vi "Source Voltage PPMU.vi"(8 "error in (no error)":errorcluster, 9 "voltage level":dbl, 10 "All Pins":string[](array[string]), 11 "Semiconductor Module Context":T1) -> (0 "error out":errorcluster, 3 "voltage measurements":dbl[][](array[numeric]))   [LabVIEW 2013]
uses:
  <vilib>/NI_TestStand_SemiconductorModule/NI_TestStand_Semiconductor_Module.lvlibp/PinMap/General/SemiconductorModuleContext.ctl
  <vilib>/NI_TestStand_SemiconductorModule/NI_TestStand_Semiconductor_Module.lvlibp/PinMap/General/NIInstrumentTypeIDs.ctl
  <vilib>/NI_TestStand_SemiconductorModule/NI_TestStand_Semiconductor_Module.lvlibp/PinMap/HSDIO/PinsToNIHSDIOSessions.vi
  <vilib>/NI_TestStand_SemiconductorModule/NI_TestStand_Semiconductor_Module.lvlibp
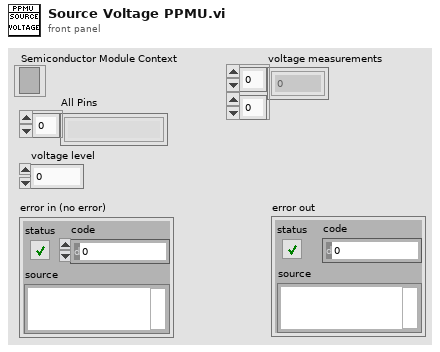
[diagram p1: front panel]
types:
  T1 = typedef "NI_TestStand_Semiconductor_Module.lvlibp/SemiconductorModuleContext.ctl" = refnum<k7>
  T2 = typedef "NI_TestStand_Semiconductor_Module.lvlibp/NIInstrumentTypeIDs.ctl" = string
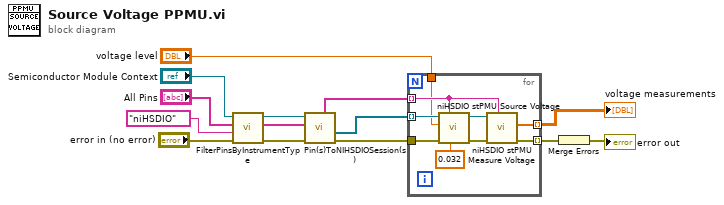
[diagram p0: block diagram]
diagram:
  n1 = call <vilib>:"FilterPinsByInstrumentType.vi"("error in (no error)"="error in (no error)", "Instrument Type Id"=T2 "niHSDIO", "Pins"="All Pins", "Semiconductor Module Context"="Semiconductor Module Context") -> ("error out"=w14:errorcluster, "Filtered Pins"=w6:string[], "Semiconductor Module Context Out"=w13:T1)  [unwired: 5 in]
  n2 = call-poly <vilib>:"Pin(s)ToNIHSDIOSession(s).vi"("error in (no error)"=w14, "Pins"=w6, "Semiconductor Module Context"=w13) -> ("error out"=w9:errorcluster, "Generation Sessions"=w8:refnum<k15>[], "Channel Lists"=w7:string[])  [unwired: 3 in, 3 out]
  n3 = for {
    tunnel: w9 -> [w23]
    tunnel: w8 -> [w22] mode=indexing
    tunnel: w7 -> [w20] mode=indexing
    tunnel: [w17] -> w3 mode=indexing
    tunnel: [w16] -> w5 mode=indexing
    tunnel: "voltage level" -> [w15]
    n4 = call <instrlib>:"niHSDIO stPMU Source Voltage.vi"("current range"=0.032, "channel list"=w20, "error in (no error)"=w23, "voltage level"=w15, "instrument handle"=w22) -> ("error out"=w18:errorcluster, "instrument handle out"=w19:refnum<k15>)  [unwired: 5 in]
    n5 = call <instrlib>:"niHSDIO stPMU Measure Voltage.vi"("channel list"=w20, "error in (no error)"=w18, "instrument handle"=w19) -> ("error out"=w16:errorcluster, "voltage measurements"=w17:dbl[])  [unwired: 6 in, 1 out]
  }
  "voltage measurements" <- w3
  n6 = Merge Errors(w5) -> (→"error out":errorcluster)
